vi "Griddy is not Finished.vi"(10 "Start Time":u32, 11 "Timeout":dbl) -> (3 "Griddy Not Finished?":bool)   [LabVIEW 2020]
uses:
  Typedefs/Manipulator State.ctl
  24b6915f-85b1-4bfc-b1f9-9b7280a96051.vi
  Framework/Robot Global Data.vi
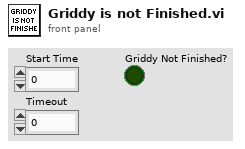
[diagram p1: front panel]
types:
  T1 = typedef "Manipulator State.ctl" = enum16{"Wrist Safety", "Cascade", "Wrist Final", "Finished"}
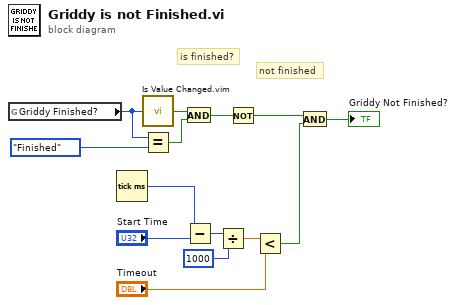
[diagram p0: block diagram]
diagram:
  # "not finished"
  # "is finished?"
  n1 = global read "Robot Global Data.vi" "Griddy Finished?"() -> (w14:T1)
  n2 = Tick Count (ms)() -> (millisecond timer value=w9:u32)
  n3 = call "Is Value Changed.vim"("value"=w14) -> ("changed or first call?"=w12:bool)
  n4 = Equal?(x=w14, y=Manipulator_State."Finished") -> (x = y?=w11:bool)
  n5 = And(x=w12, y=w11) -> (x .and. y?=w10:bool)
  n6 = Subtract(x=w9, y="Start Time") -> (x-y=w8:u32)
  n7 = Divide(x=w8, y=u32 1000) -> (x/y=w6:dbl)
  n8 = Not(x=w10) -> (.not. x?=w3:bool)
  n9 = Less?(x=w6, y="Timeout") -> (x < y?=w2:bool)
  n10 = And(x=w3, y=w2) -> (x .and. y?=→"Griddy Not Finished?":bool)
